vi "SLL DE File Looging Utility.vi"(8 "error in (no error)":errorcluster) -> (0 "error out":errorcluster)   [LabVIEW 2013]
uses:
  Controls/SLL DE File Logging Options.ctl
  DAQ Engine/Controls/SLL DE DO Command LV2Global Options.ctl
  DAQ Engine/Controls/SLL DE DAQ Global Elements.ctl
  DAQ Engine/Controls/SLL DE DAQ Global Options.ctl
  Controls/SLL DE Virtual Chart Datalog Driver Options.ctl
  DAQ Engine/Controls/SLL DE Circular Buffer Options.ctl
  DAQ Engine/Controls/SLL DE Circular Buffer Pointers List.ctl
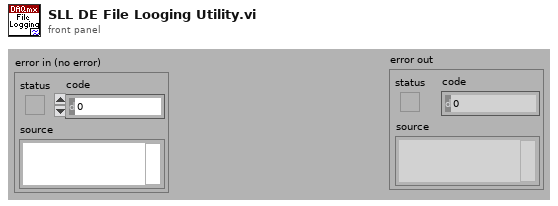
[diagram p1: front panel]
types:
  T1 = typedef "SLL DE File Logging Options.ctl" = enum16{">Initialize", ">Poll", ">Update Headings", ">Log to File", ">Stop Logging", ">Error", ">Exit"}
  T2 = typedef "SLL DE DO Command LV2Global Options.ctl" = enum16{"Init/Register Events", "Get Event Refnum", "Fire Event", "Destroy Event"}
  T3 = typedef "SLL DE DAQ Global Options.ctl" = enum16{"Init", "Write 1", "Read 1", "Write Array", "Read Array", "Clear"}
  T4 = typedef "SLL DE DAQ Global Elements.ctl" = enum16{"AI Error", "AO Error", "DI Error", "DO Error", "AI Restart", "DI Restart", "AI Running", "AO Running", "DI Running", "DO Running", "DAQ Exit?"}
  T5 = typedef "SLL DE Circular Buffer Pointers List.ctl" = enum16{"Graph Pointer", "File Log Pointer", "Pointer 3", "Pointer 4"}
  T6 = typedef "SLL DE Circular Buffer Options.ctl" = enum16{"Initialize", "Init Pointer X", "Write", "Read Single Value", "Read Pointer X (Multi Value)", "Clear Data"}
  T7 = typedef "SLL DE Virtual Chart Datalog Driver Options.ctl" = enum16{"Initialise", "Write Headings", "Write", "Check File Size", "Read", "Clear"}
  T8 = cluster{"File Logging":bool, "File - Interval b/w Samples":i32, "AI Sampling Rate (Samples/Sec)":dbl, "File Mod":i32}
  T9 = typedef "SLL DE File Logging Command List.ctl" = enum16{"Start Logging", "Stop Logging"}
  T10 = enum16{"Left Button", "Center Button", "Right Button", "Window Close"}
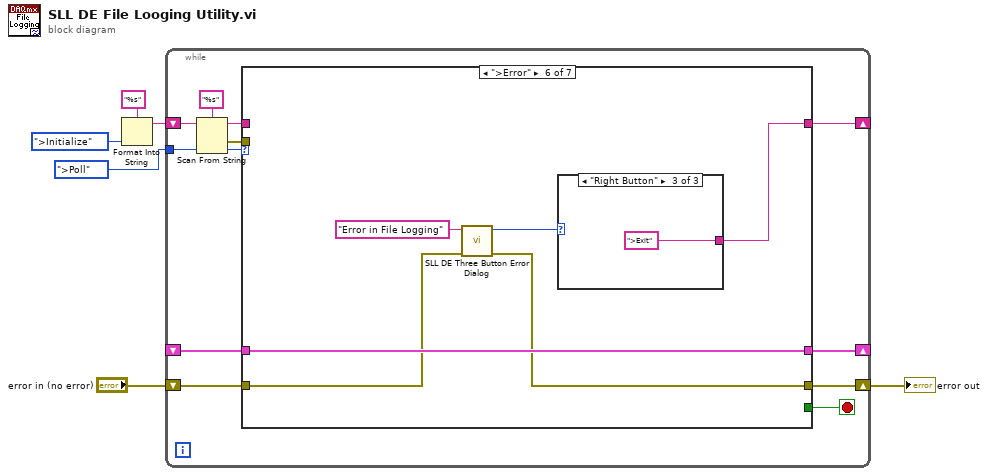
[diagram p0: block diagram]
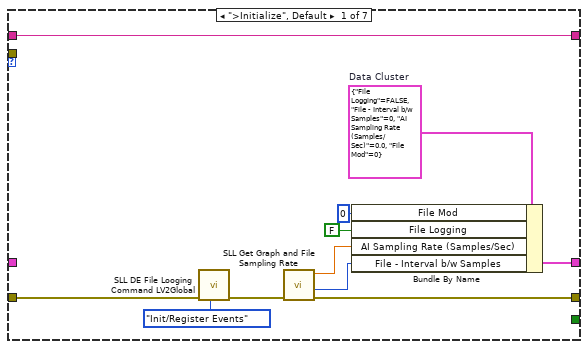
[diagram p2: hidden frame]
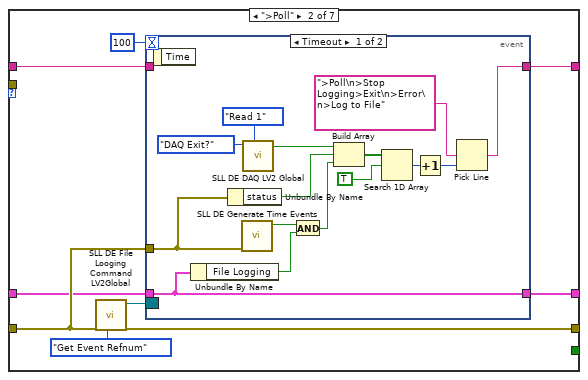
[diagram p3: hidden frame]
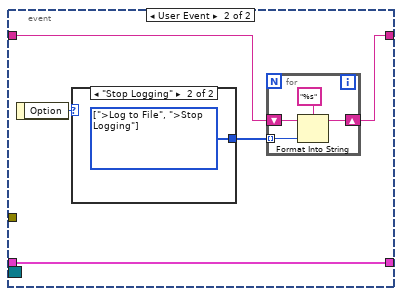
[diagram p4: hidden frame]
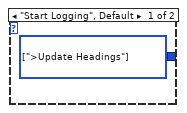
[diagram p5: hidden frame]
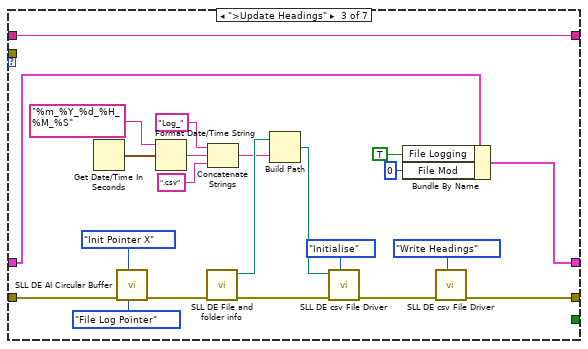
[diagram p6: hidden frame]
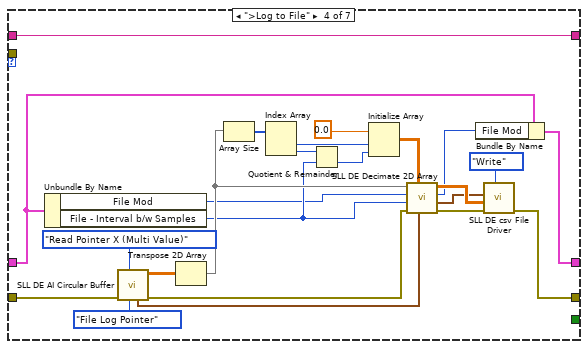
[diagram p7: hidden frame]
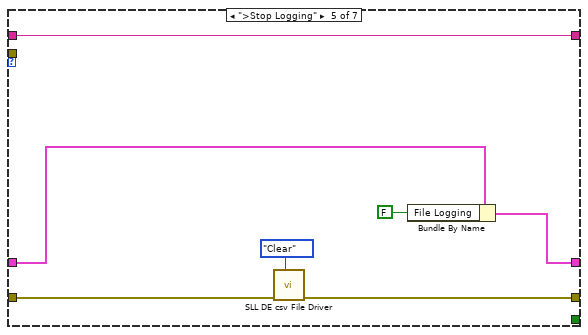
[diagram p8: hidden frame]
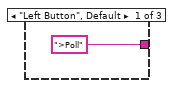
[diagram p9: hidden frame]
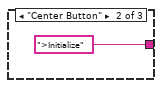
[diagram p10: hidden frame]
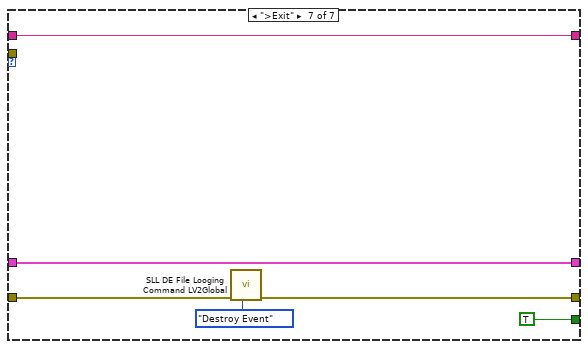
[diagram p11: hidden frame]
diagram:
  n1 = Format Into String(format string="%s", SLL_DE_File_Logging_Options.">Initialize" ("Option")) -> (resulting string=w6:string)  [unwired: 2 in, 1 out]
  n2 = while {
    tunnel: SLL_DE_File_Logging_Options.">Poll" ("Option") -> [w16]
    shift-right: [w14] -> _
    shift-left: w6 -> [w18]
    shift-right: [w10] -> w1
    shift-left: "error in (no error)" -> [w11]
    shift-right: [w9] -> _
    shift-left: _ -> [w8]
    stop <- w12 stop-if-true
    n3 = Scan From String(format string="%s", input string=w18, default 1=w16) -> (remaining string=w13:string, error out=w7:errorcluster, output 1=w15:T1)  [unwired: 2 in, 1 out]
    n4 = case shown="\">Error\"" w15 {
      tunnel: [w29 w33 w81 w105 w114 w118 w130] -> w14
      tunnel: w13 -> [w29 w38 w81 w105 w114 _ w130]
      tunnel: [_ _ _ _ _ _ TRUE] -> w12
      tunnel: w11 -> [w28 w32 w75 w108 w116 w120 w128]
      tunnel: [w25 w36 w82 w106 w115 w119 w127] -> w10
      tunnel: [w23 w30 w79 w88 w112 w123 w131] -> w9
      tunnel: w8 -> [_ w31 w80 w89 w113 w123 w131]
      tunnel: w7 -> [_ _ _ _ _ _ _]
      frame ">Initialize", Default {
        w24 = T8 {"File Logging"=FALSE, "File - Interval b/w Samples"=0, "AI Sampling Rate (Samples/Sec)"=0.0, "File Mod"=0}  # Data Cluster
        n5 = call "SLL DE File Looging Command LV2Global.vi"("Option"=SLL_DE_DO_Command_LV2Global_Options."Init/Register Events", "Error in (no error)"=w28) -> ("Error out"=w26:errorcluster)  [unwired: 8 in, 1 out]
        n6 = call "SLL Get Graph and File Sampling Rate.vi"("error in (no error)"=w26) -> ("error out"=w25:errorcluster, "File - Interval b/w Samples"=w20:i32, "AI Sampling Rate (Samples/Sec)"=w21:dbl)  [unwired: 7 in, 1 out]
        n7 = Bundle By Name(cluster=w24, "File Mod"=0, "File Logging"=FALSE, "AI Sampling Rate (Samples/Sec)"=w21, "File - Interval b/w Samples"=w20) -> (w23:T8)
      }
      frame ">Poll" {
        n8 = call "SLL DE File Looging Command LV2Global.vi"("Option"=SLL_DE_DO_Command_LV2Global_Options."Get Event Refnum", "Error in (no error)"=w32) -> ("Error out"=w36:errorcluster, "Event Registration Refnum"=w37:refnum<event-registration>)  [unwired: 1 in, 7 out]
        n9 = event shown="[0] Timeout" {
          selector: w37 -> [_ _]
          dyn-events: _ -> [_ _]
          timeout: 100 -> [_ _]
          tunnel: w38 -> [_ w56]
          tunnel: [w40 w55] -> w33
          tunnel: w32 -> [w51 _]
          tunnel: w31 -> [w50 w54]
          tunnel: [w50 w54] -> w30
          event Timeout {
            n10 = event-data() -> ()  [unwired: 2 out]
            n11 = Unbundle By Name(w50) -> ("File Logging"=w48:bool)
            n12 = Unbundle By Name(w51) -> ("status"=w46:bool)
            n13 = call "SLL DE Generate Time Events.vi"("error in (no error)"=w51) -> ("2 Mins"=w49:bool)  [unwired: 8 in, 2 out]
            n14 = call "SLL DE DAQ LV2 Global.vi"("Option"=SLL_DE_DAQ_Global_Options."Read 1", "Element"=SLL_DE_DAQ_Global_Elements."DAQ Exit?") -> ("Status Out"=w47:bool)  [unwired: 7 in, 2 out]
            n15 = And(x=w49, y=w48) -> (x .and. y?=w45:bool)
            n16 = Build Array(w47, w46, w45) -> (w44:bool[])
            n17 = Search 1D Array(1D array=w44, element=TRUE) -> (index of element=w42:i32)  [unwired: 1 in]
            n18 = Increment(x=w42) -> (x+1=w41:i32)
            n19 = Pick Line(multi-line string=">Poll\n>Stop Logging>Exit\n>Error\n>Log to File" ("format string"), line index=w41) -> (output string=w40:string)  [unwired: 1 in]
          }
          event User Event {
            n20 = event-data() -> ("Option"=w58:T9)  [unwired: 1 out]
            n21 = case shown="\"Stop Logging\"" w58 {
              tunnel: [w63 w64] -> w57
              frame "Start Logging", Default {
                w63 = T1[] [enum.">Update Headings"] items=[">Initialize", ">Poll", ">Update Headings", ">Log to File", ">Stop Logging", ">Error", ">Exit"]
              }
              frame "Stop Logging" {
                w64 = T1[] [enum.">Log to File", enum.">Stop Logging"] items=[">Initialize", ">Poll", ">Update Headings", ">Log to File", ">Stop Logging", ">Error", ">Exit"]
              }
            }
            n22 = for {
              tunnel: w57 -> [w61] mode=indexing
              shift-right: [w59] -> w55
              shift-left: w56 -> [w60]
              n23 = Format Into String(format string="%s", initial string=w60, w61) -> (resulting string=w59:string)  [unwired: 1 in, 1 out]
            }
          }
        }
      }
      frame ">Update Headings" {
        n24 = Get Date/Time In Seconds() -> (seconds since 1Jan1904=w68:timestamp)
        n25 = call "SLL DE AI Circular Buffer.vi"("Pointers"=SLL_DE_Circular_Buffer_Pointers_List."File Log Pointer", "Options"=SLL_DE_Circular_Buffer_Options."Init Pointer X" ("AI Option"), "error in (no error)"=w75) -> ("error Out"=w74:errorcluster)  [unwired: 3 in, 5 out]
        n26 = Format Date/Time String(time format string (%c)="%m_%Y_%d_%H_%M_%S", seconds (now)=w68) -> (date/time string=w72:string)  [unwired: 1 in]
        n27 = call "SLL DE File and folder info.vi"("error in (no error)"=w74) -> ("error out"=w84:errorcluster, "Report path"=w67:path)  [unwired: 5 in, 4 out]
        n28 = Concatenate Strings("Log_" ("string"), w72, ".csv" ("string")) -> (w66:string)
        n29 = Build Path(base path=w67, name or relative path=w66) -> (appended path=w65:path)
        n30 = call "SLL DE csv File Driver.vi"("Datalog Driver Cases"=SLL_DE_Virtual_Chart_Datalog_Driver_Options."Initialise", "error in(no error)"=w84, "Datalog path (use dialog)"=w65) -> ("error out"=w83:errorcluster)  [unwired: 4 in, 4 out]
        n31 = Bundle By Name(cluster=w80, "File Logging"=TRUE, "File Mod"=0) -> (w79:T8)
        n32 = call "SLL DE csv File Driver.vi"("Datalog Driver Cases"=SLL_DE_Virtual_Chart_Datalog_Driver_Options."Write Headings", "error in(no error)"=w83) -> ("error out"=w82:errorcluster)  [unwired: 5 in, 4 out]
      }
      frame ">Log to File" {
        n33 = Unbundle By Name(w89) -> ("File Mod"=w92:i32, "File - Interval b/w Samples"=w93:i32)
        n34 = call "SLL DE AI Circular Buffer.vi"("Pointers"=SLL_DE_Circular_Buffer_Pointers_List."File Log Pointer", "Options"=SLL_DE_Circular_Buffer_Options."Read Pointer X (Multi Value)" ("AI Option"), "error in (no error)"=w108) -> ("error Out"=w91:errorcluster, "Output Data"=w104:sgl[][], "Multi Time Stamp"=w94:timestamp[])  [unwired: 3 in, 3 out]
        n35 = Transpose 2D Array(2D array=w104) -> (transposed array=w97:sgl[][])
        n36 = Array Size(array=w97) -> (size(s)=w98:i32[])
        n37 = Index Array(array=w98) -> (element #1=w102:i32, element #2=w101:i32)  [unwired: 2 in]
        n38 = Quotient & Remainder(x=w101, y=w93) -> (floor(x/y)=w103:i32)  [unwired: 1 out]
        n39 = Initialize Array(sgl 0.0, w102, w103) -> (w100:sgl[][])
        n40 = call "SLL DE Decimate 2D Array.vi"("Multi Time Stamp"=w94, "Ref Array"=w100, "error in (no error)"=w91, "Decimation Rate"=w93, "Mod"=w92, "Data Array"=w97) -> ("error out"=w90:errorcluster, "Time array"=w95:timestamp[], "Mod Out"=w87:i32, "Data Array Out"=w96:sgl[][])  [unwired: 2 in]
        n41 = Bundle By Name(cluster=w89, "File Mod"=w87) -> (w88:T8)
        n42 = call "SLL DE csv File Driver.vi"("Datalog Driver Cases"=SLL_DE_Virtual_Chart_Datalog_Driver_Options."Write", "error in(no error)"=w90, "Data In"=w96, "Time Array"=w95) -> ("error out"=w106:errorcluster)  [unwired: 3 in, 4 out]
      }
      frame ">Stop Logging" {
        n43 = call "SLL DE csv File Driver.vi"("Datalog Driver Cases"=SLL_DE_Virtual_Chart_Datalog_Driver_Options."Clear", "error in(no error)"=w116) -> ("error out"=w115:errorcluster)  [unwired: 5 in, 4 out]
        n44 = Bundle By Name(cluster=w113, "File Logging"=FALSE) -> (w112:T8)
      }
      frame ">Error" {
        n45 = call "SLL DE Three Button Error Dialog.vi"("Error In"=w120, "Window Title"="Error in File Logging") -> ("Error Out"=w119:errorcluster, "Which Button?"=w122:T10)  [unwired: 8 in]
        n46 = case shown="\"Right Button\"" w122 {
          tunnel: [">Poll" ("Window Title") ">Initialize" ("Window Title") ">Exit" ("Window Title")] -> w118
          frame "Left Button", Default {
          }
          frame "Center Button" {
          }
          frame "Right Button" {
          }
        }
      }
      frame ">Exit" {
        n47 = call "SLL DE File Looging Command LV2Global.vi"("Option"=SLL_DE_DO_Command_LV2Global_Options."Destroy Event", "Error in (no error)"=w128) -> ("Error out"=w127:errorcluster)  [unwired: 8 in, 1 out]
      }
    }
  }
  "error out" <- w1
